vi "TCP - Send Initialization Command to DAQ.vi"(8 "error in (no error)":errorcluster, 11 "TCP Network Connection in":refnum<k5>) -> (0 "error out":errorcluster, 3 "TCP Network Connection out":refnum<k5>)   [LabVIEW 2021]
doc: "Send a series of commands to initialize the DAQ device.\nTurn echo on, stop any data streaming, set power state, set data format to JSON."
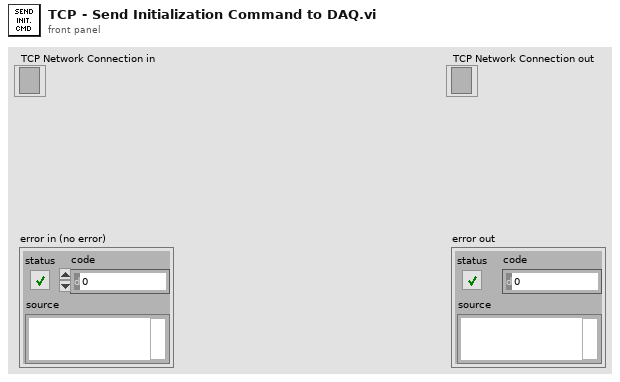
[diagram p1: front panel]
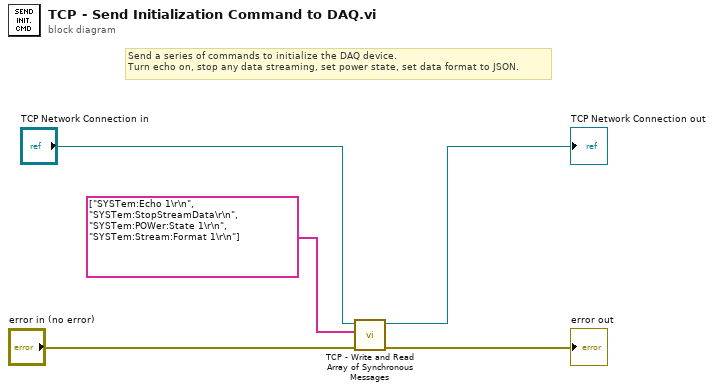
[diagram p0: block diagram]
diagram:
  # "Send a series of commands to initialize the DAQ device.\nTurn echo on, stop any data streaming, set power state, set data format to JSON."
  n1 = call "TCP - Write and Read Array of Synchronous Messages.vi"("error in"="error in (no error)", "Array of Messages to Send"=string[] ["SYSTem:Echo 1\r\n", "SYSTem:StopStreamData\r\n", "SYSTem:POWer:State 1\r\n", "SYSTem:Stream:Format 1\r\n"], "TCP Network Connection in"="TCP Network Connection in") -> ("error out"=→"error out":errorcluster, "TCP Network Connection out"=→"TCP Network Connection out":refnum<k5>)  [unwired: 6 in, 1 out]
